vi "replace_model_controls.vi"(8 "error in (no error)":errorcluster, 10 "Image File":path, 11 "Control path":path) -> (0 "error out":errorcluster, 3 "vi refnum":refnum<vi>)   [LabVIEW 2020]
doc: "Build a decision tree classifier from the training set (X, y)."
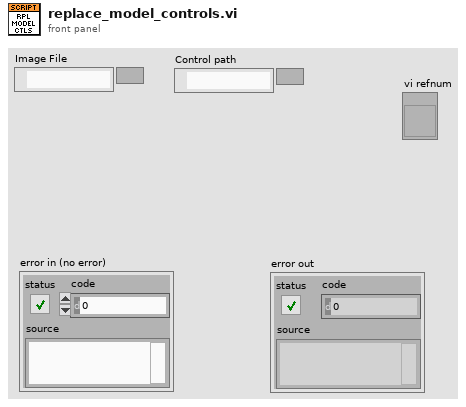
[diagram p1: front panel]
types:
  T1 = enum32{"invalid VI type", "Standard VI", "Control VI", "Global VI", "Polymorphic VI", "Configuration VI", "SubSystem", "Facade VI", "Method VI", "Statechart Diagram VI"}
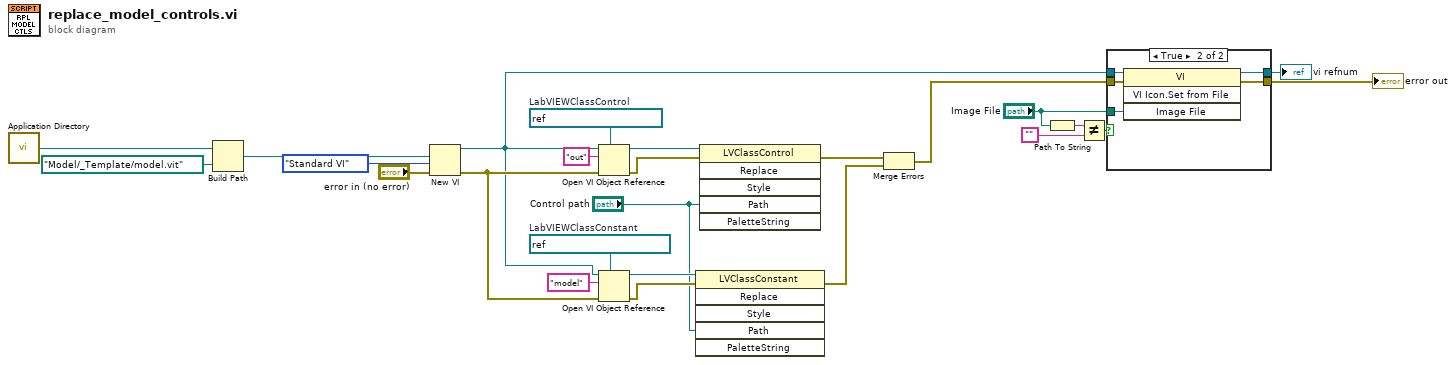
[diagram p0: block diagram]
diagram:
  w16 = refnum<vi> refnum  # LabVIEWClassConstant
  w21 = refnum<vi> refnum  # LabVIEWClassControl
  n1 = call <vilib>:"Application Directory.vi"() -> ("Application Directory"=w25:path)
  n2 = Build Path(base path=w25, name or relative path=path "Model/_Template/model.vit") -> (appended path=w23:path)
  n3 = New VI(8:"error in (no error)", 9:T1."Standard VI" ("vi type (standard vi)"), 10:w23) -> (0:w12:errorcluster, 3:w8:refnum<vi>)  [unwired: 4 in]
  n4 = Open VI Object Reference(7:w21, 8:w12, 10:"out" ("name/order"), 11:w8) -> (0:w17:errorcluster, 3:w18:refnum<vi>)
  n5 = Open VI Object Reference(7:w16, 8:w12, 10:"model" ("name/order"), 11:w8) -> (0:w13:errorcluster, 3:w14:refnum<vi>)
  n6 = invoke class="LVClassConstant" method="Replace"(reference=w14, error in=w13, "Path"="Control path") -> (error out=w10:errorcluster)  [unwired: 3 in, 5 out]
  n7 = invoke class="LVClassControl" method="Replace"(reference=w18, error in=w17, "Path"="Control path") -> (error out=w11:errorcluster)  [unwired: 3 in, 5 out]
  n8 = Merge Errors(w11, w10) -> (w7:errorcluster)
  n9 = Path To String(path="Image File") -> (string=w5:string)
  n10 = Not Equal?(x=w5, y="") -> (x != y?=w3:bool)
  n11 = case shown="True" w3 {
    tunnel: w8 -> [w27 w32]
    tunnel: w7 -> [w26 w31]
    tunnel: "Image File" -> [_ w30]
    tunnel: [w26 w29] -> w2
    tunnel: [w27 w28] -> w1
    frame False {
    }
    frame True {
      n12 = invoke class="VI" method="VI Icon.Set from File"(reference=w32, error in=w31, "Image File"=w30) -> (reference out=w28:refnum<vi>, error out=w29:errorcluster)  [unwired: 1 in, 2 out]
    }
  }
  "error out" <- w2
  "vi refnum" <- w1
